vi "hei2.vi"() -> ()   [LabVIEW 2015]
uses:
  BERTTA.dll
panel:
  in  "PORT":dbl=20.0
  out "Waveform Chart 2":dbl(graph)
  out "Waveform Chart":dbl(graph)
  in  "Heidolph 1":dbl(slide) scale=0.0..1000.0
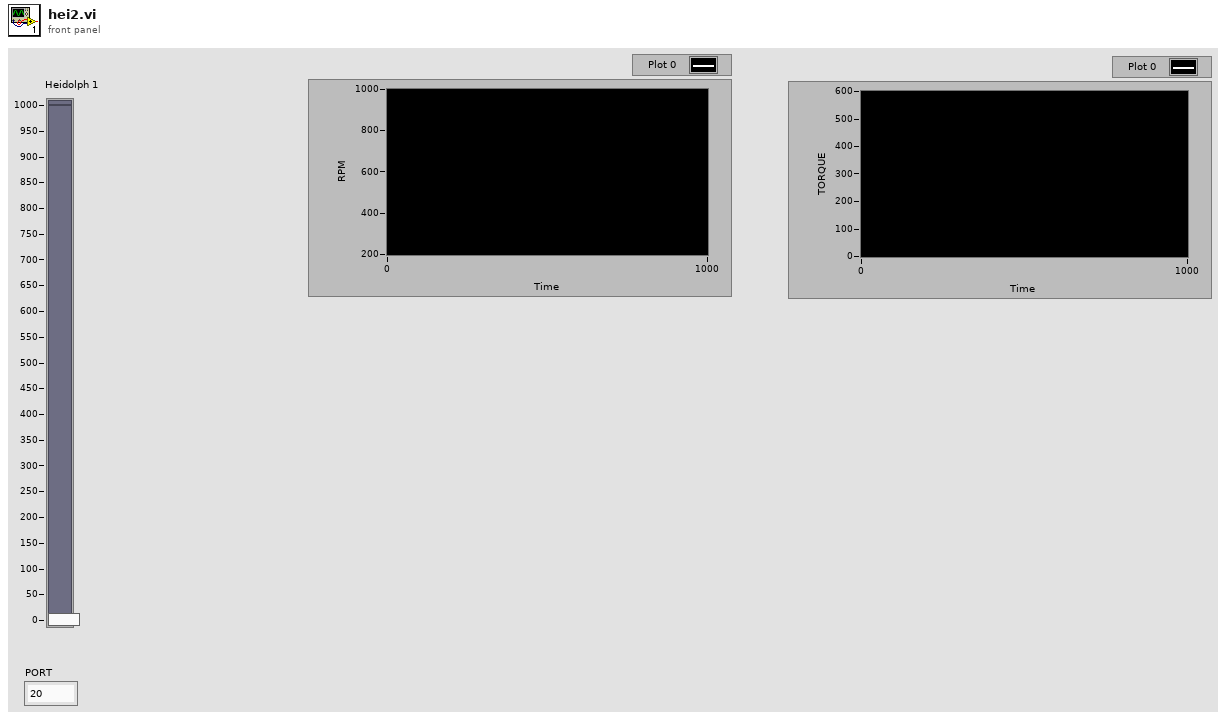
[diagram p1: front panel]
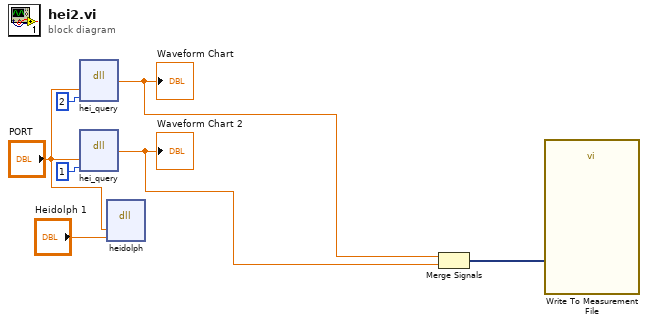
[diagram p0: block diagram]
diagram:
  n1 = dll-call lib="C:/Users/xlaraser/Documents/Visual Studio 2017/Projects/Bertta/BERTTA/Debug/BERTTA.dll" fn="hei_query"("port"="PORT", "q"=2) -> ("return type"=w3:dbl)  [unwired: 5 in, 2 out]
  "Waveform Chart" <- w3
  n2 = dll-call lib="C:/Users/xlaraser/Documents/Visual Studio 2017/Projects/Bertta/BERTTA/Debug/BERTTA.dll" fn="hei_query"("port"="PORT", "q"=1) -> ("return type"=w2:dbl)  [unwired: 5 in, 2 out]
  "Waveform Chart 2" <- w2
  n3 = dll-call lib="C:/Users/xlaraser/Documents/Visual Studio 2017/Projects/Bertta/BERTTA/Debug/BERTTA.dll" fn="heidolph"("port"="PORT", "speed"="Heidolph 1") -> ()  [unwired: 6 in, 2 out]
  n4 = Merge Signals(w3, w2) -> (w1:dynamicdata)
  n5 = call "Write To Measurement File"("Signals"=w1) -> ()  [unwired: 16 in, 3 out]
